vi "ep_Determine Parameters.vi"(8 "error in (no error)":errorcluster, 11 "system info in":refnum<class "EP System Info.lvclass">) -> (0 "error out":errorcluster, 1 "cycles per block":i32, 3 "line voltage?":bool, 5 "system info out":refnum<class "EP System Info.lvclass">)   [LabVIEW 2014, in "NI_EP_Power Quality.lvlib"]
uses:
  <vilib>/addons/Electrical Power/PQ/NI_EP_Power Quality.lvlib
  <vilib>/addons/Electrical Power/PQ/Common/Classes/System Info/EP System Info.lvclass
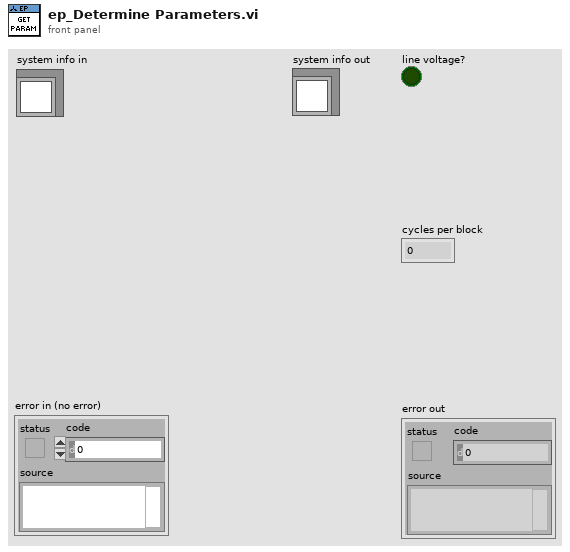
[diagram p1: front panel]
types:
  T1 = typedef "NI_EP_Power Quality.lvlib/ep_Symmetrical Component Calculation.ctl" = u16
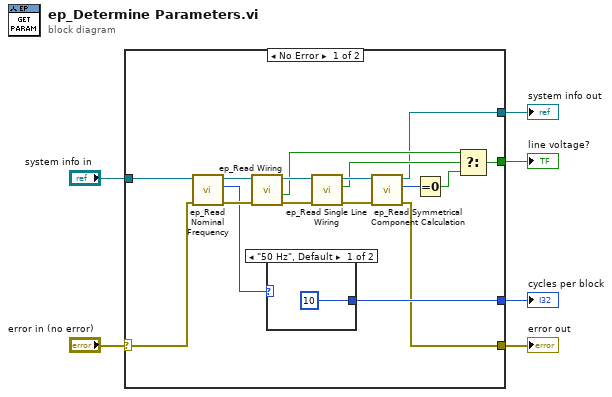
[diagram p0: block diagram]
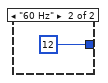
[diagram p2: hidden frame]
diagram:
  n1 = case shown="No Error" "error in (no error)" {
    selector: "error in (no error)" -> [w11 w27]
    tunnel: [w10 w27] -> w5
    tunnel: [w23 _] -> w4
    tunnel: "system info in" -> [w9 w26]
    tunnel: [w8 w26] -> w2
    tunnel: [w7 _] -> w1
    frame No Error {
      n2 = call <vilib>:"ep_Read Nominal Frequency.vi"("error in (no error)"=w11, "system info in"=w9) -> ("error out"=w13:errorcluster, "nominal frequency"=w12:enum16{"50 Hz", "60 Hz"}, "system info out"=w14:refnum<class "EP System Info.lvclass">)  [unwired: 6 in, 1 out]
      n3 = call <vilib>:"ep_Read Wiring.vi"("error in (no error)"=w13, "system info in"=w14) -> ("error out"=w16:errorcluster, "line voltage?"=w18:bool, "system info out"=w19:refnum<class "EP System Info.lvclass">)  [unwired: 6 in, 1 out]
      n4 = case shown="\"50 Hz\", Default" w12 {
        tunnel: [10 12] -> w23
        frame "50 Hz", Default {
        }
        frame "60 Hz" {
        }
      }
      n5 = call <vilib>:"ep_Read Single Line Wiring.vi"("error in (no error)"=w16, "system info in"=w19) -> ("error out"=w15:errorcluster, "single line wiring? (F)"=w17:bool, "system info out"=w20:refnum<class "EP System Info.lvclass">)  [unwired: 7 in]
      n6 = call <vilib>:"ep_Read Symmetrical Component Calculation.vi"("error in (no error)"=w15, "system info in"=w20) -> ("error out"=w10:errorcluster, "symmetrical component calculation"=w22:T1, "system info out"=w8:refnum<class "EP System Info.lvclass">)  [unwired: 7 in]
      n7 = Equal To 0?(x=w22) -> (x = 0?=w21:bool)
      n8 = Select(t=w18, s=w17, f=w21) -> (s? t:f=w7:bool)
    }
    frame Error {
    }
  }
  "error out" <- w5
  "cycles per block" <- w4
  "system info out" <- w2
  "line voltage?" <- w1
